vi "cw_2_3.vi"() -> ()   [LabVIEW 2022 SP3]
uses:
  <vilib>/numeric/Random Number (Range) I64.vi
  <vilib>/numeric/sub_Random U32.vi
panel:
  out "x > y?":bool
  in  "stop":bool
  out "discrimination level":bool
  in  "discrimination level":dbl=1.5 step=0.1
  in  "noise amplitude":dbl=0.5 step=0.1
  in  "frequency":dbl=2.0
  out "time":dbl
  out "Waveform Chart":cluster{dbl, "discrimination level":dbl}(graph)
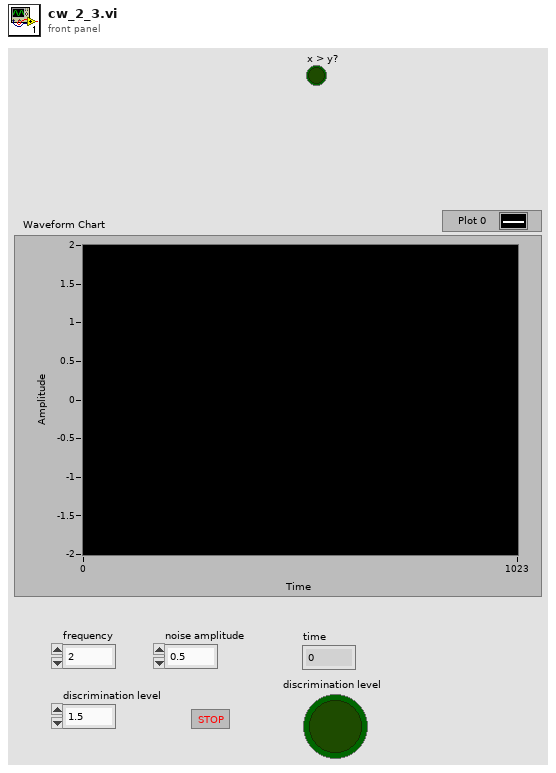
[diagram p1: front panel]
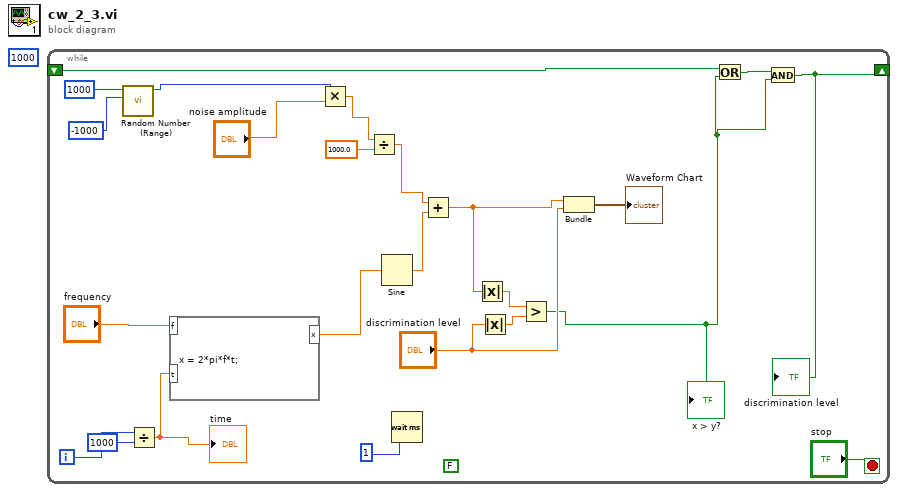
[diagram p0: block diagram]
diagram:
  (unwired) 1000
  n1 = while {
    shift-right: [w3] -> _
    shift-left: _ -> [w5]
    i -> [w24]
    stop <- "stop" stop-if-true
    (unwired) FALSE
    n2 = call-poly <vilib>:"Random Number (Range).vi"("lower bound (-100)"=i64 -1000, "upper bound (100)"=i64 1000) -> ("number"=w14:i64)  [unwired: 9 in]
    n3 = Divide(x=w24, y=1000) -> (x/y=w21:dbl)
    "time" <- w21
    n4 = formula code="x = 2*pi*f*t;"("f"="frequency", "t"=w21) -> ("x"=w22:dbl)
    n5 = Multiply(x=w14, y="noise amplitude") -> (x*y=w13:dbl)
    n6 = Divide(x=w13, y=1000.0) -> (x/y=w12:dbl)
    n7 = Sine(x=w22) -> (sin(x)=w17:dbl)
    n8 = Wait (ms)(milliseconds to wait=u32 1) -> ()  [unwired: 1 out]
    n9 = Add(x=w12, y=w17) -> (x+y=w9:dbl)
    n10 = Absolute Value(x=w9) -> (abs(x)=w7:dbl)
    n11 = Absolute Value(x="discrimination level") -> (abs(x)=w6:dbl)
    n12 = Greater?(x=w7, y=w6) -> (0:w1:bool)
    "x > y?" <- w1
    n13 = Bundle(w9, "discrimination level"="discrimination level") -> (→"Waveform Chart":cluster{dbl, "discrimination level":dbl})  [unwired: 1 in]
    n14 = Or(x=w5, y=w1) -> (x .or. y?=w4:bool)
    n15 = And(x=w4, y=w1) -> (x .and. y?=w3:bool)
    "discrimination level" <- w3
  }
